vi "getPhaseMeasurement.vi"(8 "error in (no error)":errorcluster, 9 "Source 2":string, 10 "Source 1":string, 11 "ScopeKeysight in":refnum<class "ScopeKeysight.lvclass">) -> (0 "error out":errorcluster, 2 "Numeric":dbl, 3 "ScopeKeysight out":refnum<class "ScopeKeysight.lvclass">)   [LabVIEW 2023, in "ScopeKeysight.lvclass"]
doc: "<b>Author:</b> Wolfgang\n<b>Descritpion:</b> Measure the phase shift between two sources."
uses:
  ScopeKeysight.lvclass
  ScopeKeysight.lvclass/ScopeKeysight.ctl
  Driver/Public/Data/Read Measurement (Current Value).vi
  Driver/Keysight-DSQx3014T.lvlib
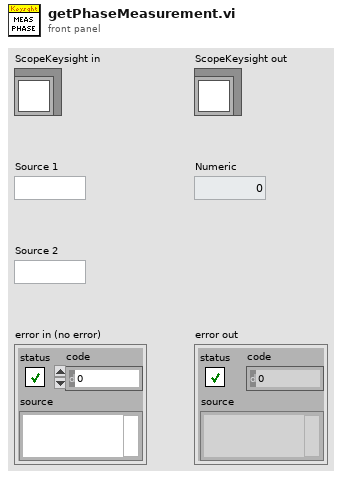
[diagram p1: front panel]
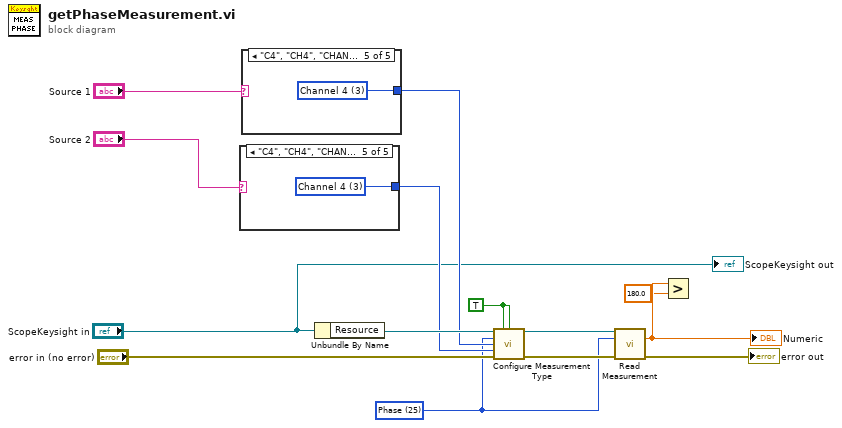
[diagram p0: block diagram]
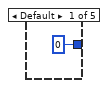
[diagram p2: hidden frame]
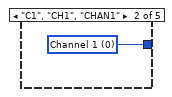
[diagram p3: hidden frame]
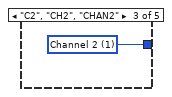
[diagram p4: hidden frame]
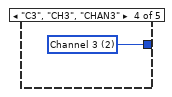
[diagram p5: hidden frame]
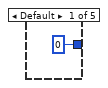
[diagram p6: hidden frame]
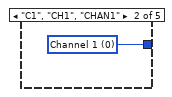
[diagram p7: hidden frame]
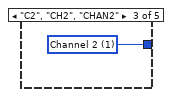
[diagram p8: hidden frame]
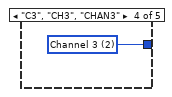
[diagram p9: hidden frame]
diagram:
  w5 = 25 items=["Peak-Peak", "Maximum", "Mimimum", "Amplitude", "Top", "Base", "Overshoot", "Preshoot", "Average - N Cycles", "Average - Full Screen", "DC RMS - N Cycles", "DC RMS - Full Screen", "AC RMS - N Cycles", "AC RMS - Full Screen (Std Dev)", "Ratio", "Period", "Frequency", "Counter", "+Width", "-Width", "Burst Width", "Duty Cycle", "Rise Time", "Fall Time", "Delay", "Phase", "X minY", "X maxY", "Positive Pulse Count", "Negative Pulse Count", "Raising Edge Count", "Falling Edge Count", "Area - N Cycle", "Area - Full Screen", "Bit Rate", "Negtive Duty Cycle", "Standard Deviation"] ("Measurement Type (0: Peak-Peak)")
  w10 = TRUE ("Enable Clear (F: Disable)")
  n1 = case shown="\"C4\", \"CH4\", \"CHAN4\"" "Source 2" {
    tunnel: [0 ("Channel Name (0: Channel 1)") w16 w17 w18 w19] -> w6
    frame Default {
    }
    frame "C1", "CH1", "CHAN1" {
      w16 = 0 items=["Channel 1", "Channel 2", "Channel 3", "Channel 4"] ("Channel Name (0: Channel 1)")
    }
    frame "C2", "CH2", "CHAN2" {
      w17 = 1 items=["Channel 1", "Channel 2", "Channel 3", "Channel 4"] ("Channel Name (0: Channel 1)")
    }
    frame "C3", "CH3", "CHAN3" {
      w18 = 2 items=["Channel 1", "Channel 2", "Channel 3", "Channel 4"] ("Channel Name (0: Channel 1)")
    }
    frame "C4", "CH4", "CHAN4" {
      w19 = 3 items=["Channel 1", "Channel 2", "Channel 3", "Channel 4"] ("Channel Name (0: Channel 1)")
    }
  }
  n2 = case shown="\"C4\", \"CH4\", \"CHAN4\"" "Source 1" {
    tunnel: [0 ("Channel Name (0: Channel 1)") w21 w22 w23 w24] -> w12
    frame Default {
    }
    frame "C1", "CH1", "CHAN1" {
      w21 = 0 items=["Channel 1", "Channel 2", "Channel 3", "Channel 4"] ("Channel Name (0: Channel 1)")
    }
    frame "C2", "CH2", "CHAN2" {
      w22 = 1 items=["Channel 1", "Channel 2", "Channel 3", "Channel 4"] ("Channel Name (0: Channel 1)")
    }
    frame "C3", "CH3", "CHAN3" {
      w23 = 2 items=["Channel 1", "Channel 2", "Channel 3", "Channel 4"] ("Channel Name (0: Channel 1)")
    }
    frame "C4", "CH4", "CHAN4" {
      w24 = 3 items=["Channel 1", "Channel 2", "Channel 3", "Channel 4"] ("Channel Name (0: Channel 1)")
    }
  }
  n3 = Unbundle By Name("ScopeKeysight in") -> ("Resource"=w14:refnum<visa-resource-name>)
  n4 = call "Configure Measurement Type.vi"("VISA resource name"=w14, "Enable Clear (F: Disable)"=w10, "Enable Statistics Reset (F: Disable)"=w10, "Measurement Type (0: Peak-Peak)"=w5, "Measurement Source 1 (0: Channel 1)"=w12, "Measurement Source 2 (1: Channel 2)"=w6, "error in (no error)"="error in (no error)") -> ("VISA resource name out"=w13:refnum<visa-resource-name>, "error out"=w11:errorcluster)  [unwired: 7 in]
  n5 = call-poly "Read Measurement.vi"("VISA resource name"=w13, "Measurement Type (0: Peak-Peak)"=w5, "error in (no error)"=w11) -> ("Result Value"=w2:dbl, "error out"=→"error out":errorcluster)  [unwired: 10 in, 1 out]
  "Numeric" <- w2
  n6 = Greater?(x=w2, y=180.0) -> ()  [unwired: 1 out]
  "ScopeKeysight out" <- "ScopeKeysight in"
